vi "ZE_Recorder_ChoseTempRTDParam.vi"(8 "error in (no error)":errorcluster, 11 "Refnum in":refnum<k21>) -> (0 "error out":errorcluster, 3 "Refnum out":refnum<k21>)   [LabVIEW 2025, in "ZE_Recorder.lvlib"]
doc: "ZE_Recorder_ChoseTempRTDParam.vi\n----------------------------------------------\n\n\nInputs:\n---------------------\n- error in (no error) : Cluster; \n- Refnum in : Refnum; \n\nOutputs:\n---------------------\n- error out : Cluster; \n- Refnum out : Refnum; \n\n----------------------------------------------\n22.05.2017\nZühlke Engineering AG\nCH-8952 Schlieren\nwww.zuehlke.com"
uses:
  ZE_Recorder.lvlib
  <resource>/objmgr/daqmx.rc
panel:
  in  "Parameter C":dbl=1.0
  in  "Parameter B":dbl=1.0
  in  "Parameter A":dbl=1.0
  in  "Config OK":bool
  # "Please set the custom RTD \nParameters according to the\nCallendar-Van Dusen equation"
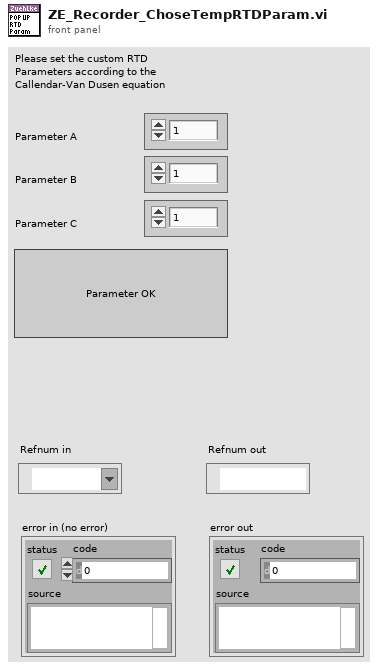
[diagram p1: front panel]
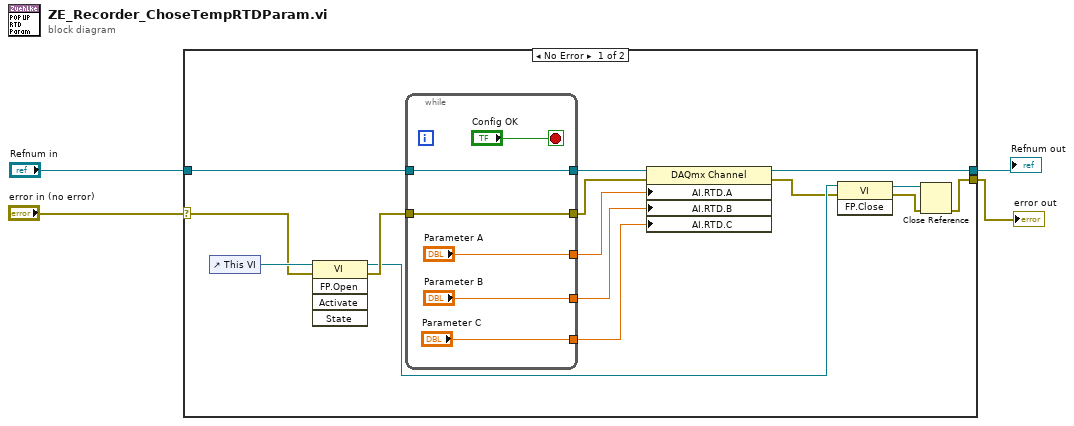
[diagram p0: block diagram]
diagram:
  n1 = case shown="No Error" "error in (no error)" {
    selector: "error in (no error)" -> [w11 w27]
    tunnel: [w7 w27] -> w4
    tunnel: [w19 w26] -> w3
    tunnel: "Refnum in" -> [w18 w26]
    frame No Error {
      n2 = control-ref of="This VI"() -> (w12:refnum<vi>)
      n3 = invoke class="VI" method="FP.Open"(reference=w12, error in=w11) -> (reference out=w9:refnum<vi>, error out=w10:errorcluster)  [unwired: 3 in, 3 out]
      n4 = while {
        tunnel: w18 -> [w21]
        tunnel: w10 -> [w20]
        tunnel: ["Parameter A"] -> w15
        tunnel: ["Parameter B"] -> w14
        tunnel: ["Parameter C"] -> w13
        tunnel: [w21] -> w17
        tunnel: [w20] -> w16
        stop <- "Config OK" stop-if-true
      }
      n5 = property class="DAQmx Channel"(reference=w17, error in=w16, "AI.RTD.A"=w15, "AI.RTD.B"=w14, "AI.RTD.C"=w13) -> (reference out=w19:refnum<k21>, error out=w8:errorcluster)
      n6 = invoke class="VI" method="FP.Close"(reference=w9, error in=w8) -> (reference out=w5:refnum<vi>, error out=w6:errorcluster)  [unwired: 1 in, 1 out]
      n7 = Close Reference(reference=w5, error in (no error)=w6) -> (error out=w7:errorcluster)
    }
    frame Error {
    }
  }
  "error out" <- w4
  "Refnum out" <- w3
